vi "old leader.vi"   [LabVIEW 2016]
uses:
  <vilib>/NXT/Block Support/NXT_OutputPort.ctl
  <vilib>/NXT/Block Support/NXT_InputPort.ctl
  <vilib>/NXT/Block Support/NXT_TimerIndex.ctl
  <vilib>/NXT/Dual Mode Library/Motors/ResetMotor.vi
  <vilib>/NXT/Dual Mode Library/Sensors/Reset_Timer.vi
  <vilib>/NXT/Dual Mode Library/Sensors/EV3_Color_Reflect.vi
  <vilib>/NXT/Dual Mode Library/Display/drawNumber_float.vi
  <vilib>/NXT/Dual Mode Library/Sensors/Touch_Pressed.vi
  <vilib>/NXT/Dual Mode Library/Display/drawText.vi
  <vilib>/NXT/Dual Mode Library/Sensors/Read_Timer.vi
  <vilib>/NXT/Dual Mode Library/Display/drawNumber.vi
  <vilib>/NXT/Dual Mode Library/Motors/Rotation.vi
  <vilib>/NXT/NXTIO Xnodes/NXTIONodeSubVIs/NXTMoveMotors.vi
  <vilib>/NXT/Dual Mode Library/Display/drawText_Right.vi
  <vilib>/NXT/NXTIO Xnodes/NXTIONodeSubVIs/NXTStopMotors.vi
  <vilib>/NXT/Subs/LVHSConnector.ctl
  <vilib>/NXT/NXTIO Xnodes/AddressXNode/NXTIOAddress.xnode
  <vilib>/NXT/NXTIO Xnodes/NXTIOXNode/NXTIO.xnode
  <vilib>/NXT/LegoClasses/BrickReference/BrickReference.lvclass
types:
  T1 = typedef "LVHSConnector.ctl" = refnum<class "BrickReference.lvclass">
  T2 = typedef "NXT_InputPort.ctl" = u32
  T3 = typedef "NXT_OutputPort.ctl" = u8
  T4 = typedef "NXT_TimerIndex.ctl" = u8
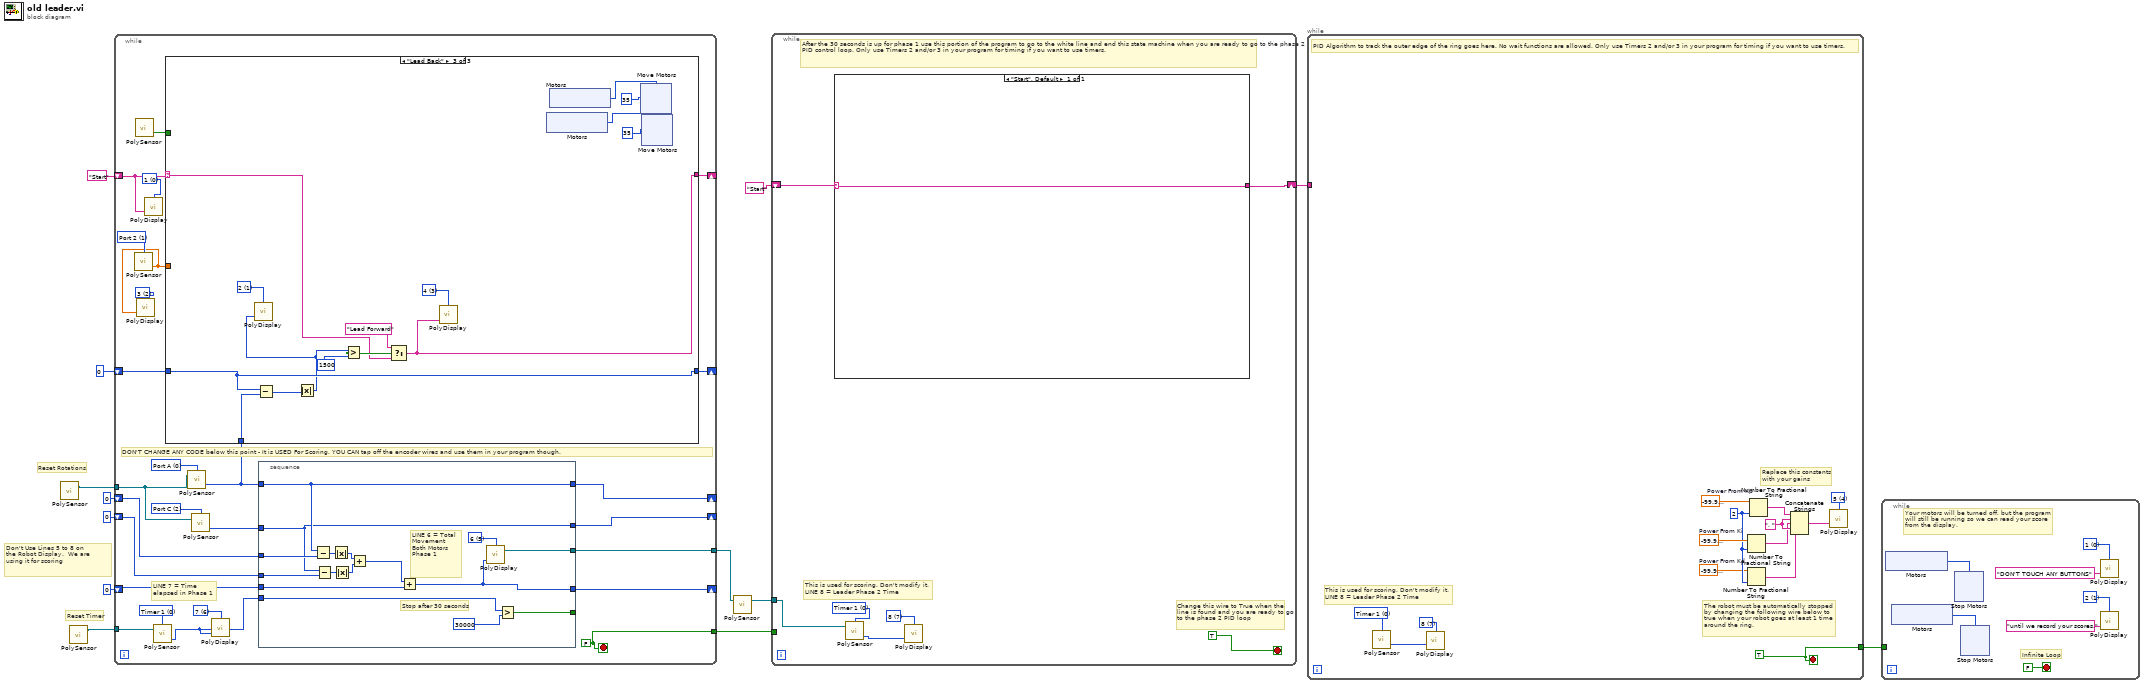
[diagram p0: block diagram]
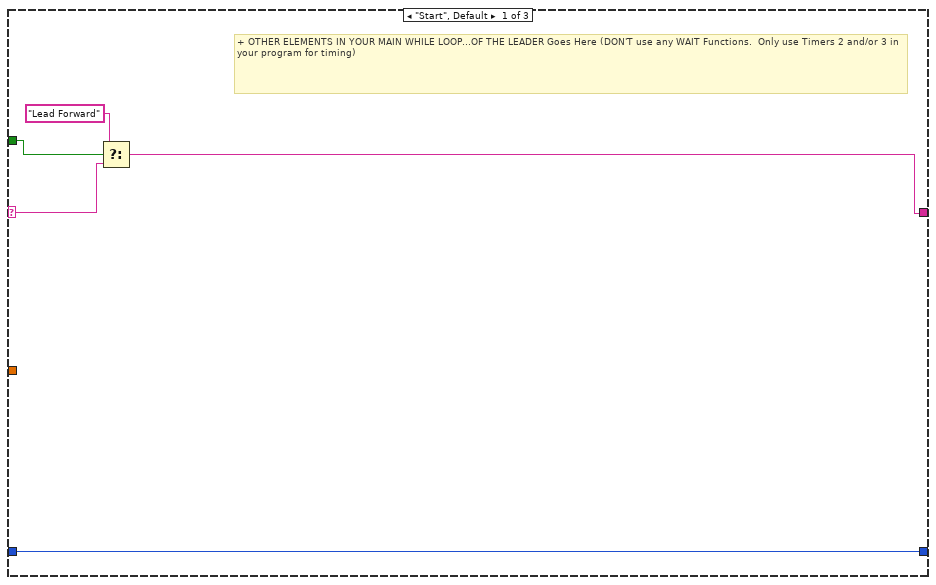
[diagram p2: hidden frame]
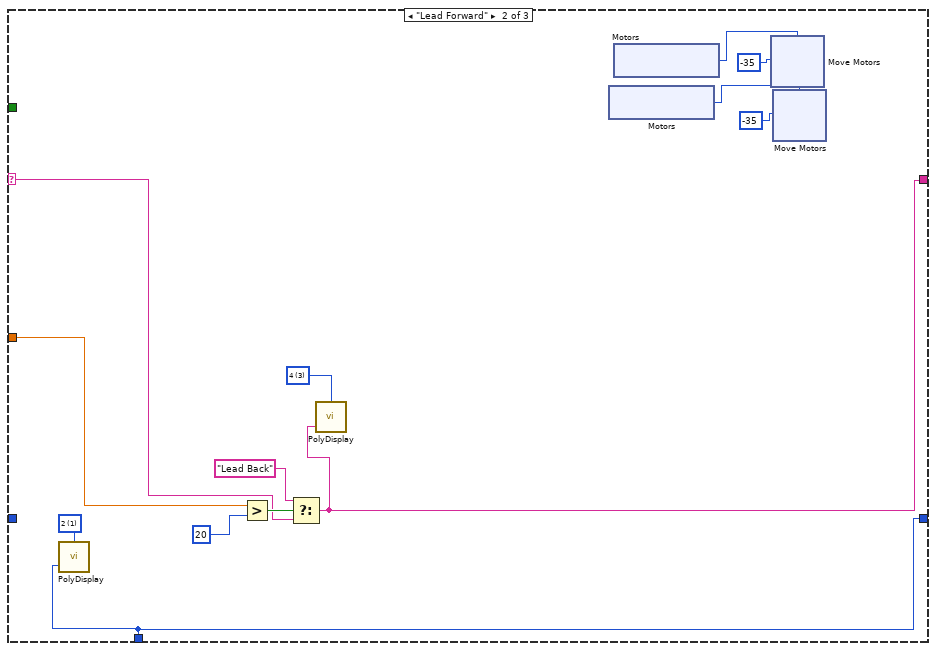
[diagram p3: hidden frame]
diagram:
  # "Don't Use Lines 5 to 8 on\nthe Robot Display.  We are \nusing it for scoring"
  # "Reset Timer"
  # "Reset Rotations"
  n1 = call-poly <vilib>:"PolySensor.vi"() -> ("NXT/EV3"=w9:T1)  [unwired: 4 in]
  n2 = call-poly <vilib>:"PolySensor.vi"() -> ("NXT/EV3"=w8:T1)  [unwired: 4 in]
  n3 = while {
    tunnel: w9 -> [w39]
    shift-right: [w34] -> _
    shift-left: 0 ("Angle of Rotation") -> [w36]
    shift-right: [w33] -> _
    shift-left: 0 ("Angle of Rotation") -> [w35]
    shift-right: [w37] -> _
    shift-left: 0 -> [w38]
    tunnel: w8 -> [w30]
    tunnel: [w14] -> w6
    shift-right: [w32] -> _
    shift-left: "Start" -> [w20]
    tunnel: [w25] -> w5
    shift-right: [w17] -> _
    shift-left: 0 -> [w18]
    stop <- w14 stop-if-true
    w14 = FALSE
    w15 = i16 2 items=["1", "2", "3", "4", "5", "6", "7", "8", "9", "10", "11", "12"] ("Line")
    w19 = T2 1 items=["Port 1", "Port 2", "Port 3", "Port 4"] ("Port (Port 1)")
    w21 = i16 0 items=["1", "2", "3", "4", "5", "6", "7", "8", "9", "10", "11", "12"] ("Line")
    w27 = i16 6 items=["1", "2", "3", "4", "5", "6", "7", "8", "9", "10", "11", "12"] ("Line")
    w28 = T3 0 items=["Port A", "Port B", "Port C", "Port D"] ("Port (Port A)")
    w29 = T3 2 items=["Port A", "Port B", "Port C", "Port D"] ("Port (Port A)")
    w31 = T4 0 items=["Timer 1", "Timer 2", "Timer 3"] ("Timer (Timer 1)")
    # "DON'T CHANGE ANY CODE below this point - It is USED For Scoring. YOU CAN tap off the encoder wires and use them in your program though."
    # "LINE 7 = Time elapsed in Phase 1"
    n4 = call-poly <vilib>:"PolySensor.vi"("Port (Port 1)"=w19) -> ("Scaled Value"=w16:sgl)  [unwired: 2 in, 1 out]
    n5 = call-poly <vilib>:"PolySensor.vi"() -> ("Yes / No"=w24:bool)  [unwired: 3 in, 1 out]
    n6 = call-poly <vilib>:"PolyDisplay.vi"("number"=w16, "Line"=w15) -> ()  [unwired: 2 in, 1 out]
    n7 = call-poly <vilib>:"PolyDisplay.vi"("Text"=w20, "Line"=w21) -> ()  [unwired: 2 in, 1 out]
    n8 = call-poly <vilib>:"PolySensor.vi"("NXT/EV3"=w30, "Timer (Timer 1)"=w31) -> ("Value (msec)"=w26:u32)  [unwired: 1 in, 1 out]
    n9 = call-poly <vilib>:"PolySensor.vi"("NXT/EV3"=w39, "Port (Port A)"=w28) -> ("Angle of Rotation"=w23:i32)  [unwired: 1 in, 1 out]
    n10 = case shown="\"Lead Back\"" w20 {
      selector: w20 -> [w41 w47 w77]
      tunnel: [w43 w48 w81] -> w32
      tunnel: w24 -> [w44 _ _]
      tunnel: w23 -> [_ w45 w78]
      tunnel: w18 -> [w40 _ w76]
      tunnel: w16 -> [_ w46 _]
      tunnel: [w40 w45 w76] -> w17
      frame "Start", Default {
        # "+ OTHER ELEMENTS IN YOUR MAIN WHILE LOOP...OF THE LEADER Goes Here (DON'T use any WAIT Functions.  Only use Timers 2 and/or 3 in your program for timing)"
        n11 = Select(t="Lead Forward", s=w44, f=w41) -> (s? t:f=w43:string)
      }
      frame "Lead Forward" {
        w50 = i16 3 items=["1", "2", "3", "4", "5", "6", "7", "8", "9", "10", "11", "12"] ("Line")
        w56 = i16 1 items=["1", "2", "3", "4", "5", "6", "7", "8", "9", "10", "11", "12"] ("Line")
        n12 = call-poly <vilib>:"PolyDisplay.vi"("number"=w45, "Line"=w56) -> ()  [unwired: 2 in, 1 out]
        n13 = Greater?(x=w46, y=20) -> (0:w49:bool)
        n14 = Select(t="Lead Back", s=w49, f=w47) -> (s? t:f=w48:string)
        n15 = call-poly <vilib>:"PolyDisplay.vi"("Text"=w48, "Line"=w50) -> ()  [unwired: 2 in, 1 out]
        n16 = xnode "Motors"() -> ("Motor"=w55:T3)
        n17 = xnode "Motors"() -> ("Motor"=w52:T3)
        n18 = xnode "Move Motors"("Power/Speed 1"=-35, "Motors"=w52) -> ()  [unwired: 1 in, 1 out]
        n19 = xnode "Move Motors"("Power/Speed 1"=-35, "Motors"=w55) -> ()  [unwired: 1 in, 1 out]
      }
      frame "Lead Back" {
        w82 = i16 3 items=["1", "2", "3", "4", "5", "6", "7", "8", "9", "10", "11", "12"] ("Line")
        w87 = i16 1 items=["1", "2", "3", "4", "5", "6", "7", "8", "9", "10", "11", "12"] ("Line")
        n20 = Subtract(x=w76, y=w78) -> (x-y=w75:i32)
        n21 = Absolute Value(x=w75) -> (abs(x)=w74:i32)
        n22 = call-poly <vilib>:"PolyDisplay.vi"("number"=w74, "Line"=w87) -> ()  [unwired: 2 in, 1 out]
        n23 = Greater?(x=w74, y=1500) -> (0:w79:bool)
        n24 = Select(t="Lead Forward", s=w79, f=w77) -> (s? t:f=w81:string)
        n25 = call-poly <vilib>:"PolyDisplay.vi"("Text"=w81, "Line"=w82) -> ()  [unwired: 2 in, 1 out]
        n26 = xnode "Motors"() -> ("Motor"=w86:T3)
        n27 = xnode "Motors"() -> ("Motor"=w84:T3)
        n28 = xnode "Move Motors"("Power/Speed 1"=35, "Motors"=w84) -> ()  [unwired: 1 in, 1 out]
        n29 = xnode "Move Motors"("Power/Speed 1"=35, "Motors"=w86) -> ()  [unwired: 1 in, 1 out]
      }
    }
    n30 = call-poly <vilib>:"PolySensor.vi"("NXT/EV3"=w39, "Port (Port A)"=w29) -> ("Angle of Rotation"=w22:i32)  [unwired: 1 in, 1 out]
    n31 = call-poly <vilib>:"PolyDisplay.vi"("number"=w26, "Line"=w27) -> ()  [unwired: 2 in, 1 out]
    n32 = stacked-sequence {
      tunnel: w38 -> [w120]
      tunnel: [w107] -> w37
      tunnel: w26 -> [w118]
      tunnel: [w117] -> _
      tunnel: w23 -> [w110]
      tunnel: w22 -> [w109]
      tunnel: w36 -> [w112]
      tunnel: w35 -> [w111]
      tunnel: [w110] -> w34
      tunnel: [w109] -> w33
      tunnel: [w105] -> w25
      frame #0 {
        w106 = i16 5 items=["1", "2", "3", "4", "5", "6", "7", "8", "9", "10", "11", "12"] ("Line")
        # "LINE 6 = Total\nMovement\nBoth Motors\nPhase 1"
        # "Stop after 30 seconds"
        n33 = Subtract(x=w110, y=w112) -> (x-y=w116:i32)
        n34 = Subtract(x=w109, y=w111) -> (x-y=w115:i32)
        n35 = Absolute Value(x=w116) -> (abs(x)=w114:i32)
        n36 = Absolute Value(x=w115) -> (abs(x)=w113:i32)
        n37 = Add(x=w114, y=w113) -> (x+y=w108:i32)
        n38 = Add(x=w108, y=w120) -> (x+y=w107:i32)
        n39 = call-poly <vilib>:"PolyDisplay.vi"("number"=w107, "Line"=w106) -> ("NXT/EV3"=w105:T1)  [unwired: 2 in]
        n40 = Greater?(x=w118, y=u32 30000 ("Value (msec)")) -> (0:w117:bool)
      }
    }
  }
  n41 = call-poly <vilib>:"PolySensor.vi"("NXT/EV3"=w5) -> ("NXT/EV3"=w4:T1)  [unwired: 3 in]
  n42 = while {
    shift-right: [w126] -> w3
    shift-left: "Start" -> [w127]
    tunnel: w6 -> [_]
    tunnel: w4 -> [w122]
    stop <- TRUE stop-if-true
    w124 = i16 7 items=["1", "2", "3", "4", "5", "6", "7", "8", "9", "10", "11", "12"] ("Line")
    w125 = T4 0 items=["Timer 1", "Timer 2", "Timer 3"] ("Timer (Timer 1)")
    # "This is used for scoring. Don't modify it.\nLINE 8 = Leader Phase 2 Time"
    # "Change this wire to True when the line is found and you are ready to go to the phase 2 PID loop"
    # "After the 30 seconds is up for phase 1 use this portion of the program to go to the white line and end this state machine when you are ready to go to the phase 2 PID control loop. Only use Timers 2 and/or 3 in your program for timing if you want to use timers."
    n43 = case shown="\"Start\", Default" w127 {
      selector: w127 -> [w128]
      tunnel: [w128] -> w126
      frame "Start", Default {
      }
    }
    n44 = call-poly <vilib>:"PolySensor.vi"("NXT/EV3"=w122, "Timer (Timer 1)"=w125) -> ("Value (msec)"=w123:u32)  [unwired: 1 in, 1 out]
    n45 = call-poly <vilib>:"PolyDisplay.vi"("number"=w123, "Line"=w124) -> ()  [unwired: 2 in, 1 out]
  }
  n46 = while {
    tunnel: [w139] -> w2
    tunnel: w3 -> [_]
    stop <- w139 stop-if-true
    w132 = ", " ("string")
    w135 = i16 2 ("precision (6)")
    w134 = sgl -99.9  # Power From Kd
    w136 = sgl -99.9  # Power From Ki
    w137 = sgl -99.9  # Power From Kp
    w138 = i16 4 items=["1", "2", "3", "4", "5", "6", "7", "8", "9", "10", "11", "12"] ("Line")
    w139 = TRUE
    w140 = i16 7 items=["1", "2", "3", "4", "5", "6", "7", "8", "9", "10", "11", "12"] ("Line")
    w142 = T4 0 items=["Timer 1", "Timer 2", "Timer 3"] ("Timer (Timer 1)")
    # "Replace this constants\nwith your gains"
    # "This is used for scoring. Don't modify it.\nLINE 8 = Leader Phase 2 Time"
    # "The robot must be automatically stopped\nby changing the following wire below to\ntrue when your robot goes at least 1 time\naround the ring."
    # "PID Algorithm to track the outer edge of the ring goes here. No wait functions are allowed. Only use Timers 2 and/or 3 in your program for timing if you want to use timers."
    n47 = call-poly <vilib>:"PolySensor.vi"("Timer (Timer 1)"=w142) -> ("Value (msec)"=w141:u32)  [unwired: 2 in, 1 out]
    n48 = call-poly <vilib>:"PolyDisplay.vi"("number"=w141, "Line"=w140) -> ()  [unwired: 2 in, 1 out]
    n49 = Number To Fractional String(number=w136, precision (6)=w135) -> (F-format string=w131:string)  [unwired: 2 in]
    n50 = Number To Fractional String(number=w134, precision (6)=w135) -> (F-format string=w130:string)  [unwired: 2 in]
    n51 = Number To Fractional String(number=w137, precision (6)=w135) -> (F-format string=w133:string)  [unwired: 2 in]
    n52 = Concatenate Strings(w133, w132, w131, w132, w130) -> (w129:string)
    n53 = call-poly <vilib>:"PolyDisplay.vi"("Text"=w129, "Line"=w138) -> ()  [unwired: 2 in, 1 out]
  }
  n54 = while {
    tunnel: w2 -> [_]
    stop <- FALSE stop-if-true
    w146 = i16 1 items=["1", "2", "3", "4", "5", "6", "7", "8", "9", "10", "11", "12"] ("Line")
    w145 = i16 0 items=["1", "2", "3", "4", "5", "6", "7", "8", "9", "10", "11", "12"] ("Line")
    # "Your motors will be turned off, but the program\nwill still be running so we can read your score\nfrom the display."
    # "Infinite Loop"
    n55 = xnode "Motors"() -> ("Motor"=w148:T3)
    n56 = xnode "Motors"() -> ("Motor"=w147:T3)
    n57 = xnode "Stop Motors"("Motors"=w148) -> ()  [unwired: 1 in, 1 out]
    n58 = xnode "Stop Motors"("Motors"=w147) -> ()  [unwired: 1 in, 1 out]
    n59 = call-poly <vilib>:"PolyDisplay.vi"("Text"="DON'T TOUCH ANY BUTTONS", "Line"=w145) -> ()  [unwired: 2 in, 1 out]
    n60 = call-poly <vilib>:"PolyDisplay.vi"("Text"="until we record your scores.", "Line"=w146) -> ()  [unwired: 2 in, 1 out]
  }
